vi "Write fsync.vi"(8 "error in (no error)":errorcluster, 10 "enable fsync":bool, 11 "session in":refnum<class "Session.lvclass">) -> (0 "error out":errorcluster, 3 "session out":refnum<class "Session.lvclass">)   [LabVIEW 2020, in "NI_SFTP.lvlib" / "Session.lvclass"]
doc: "Sets whether file data is flushed to disk after successful download or upload."
uses:
  <vilib>/net/SFTP/Session/Session.lvclass
  <vilib>/net/SFTP/Session/Session.lvclass/Session.ctl
  <vilib>/net/SFTP/Session/Is Connected.vi
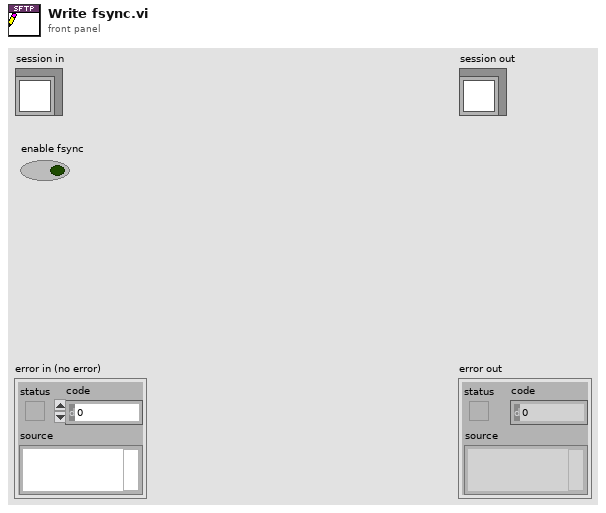
[diagram p1: front panel]
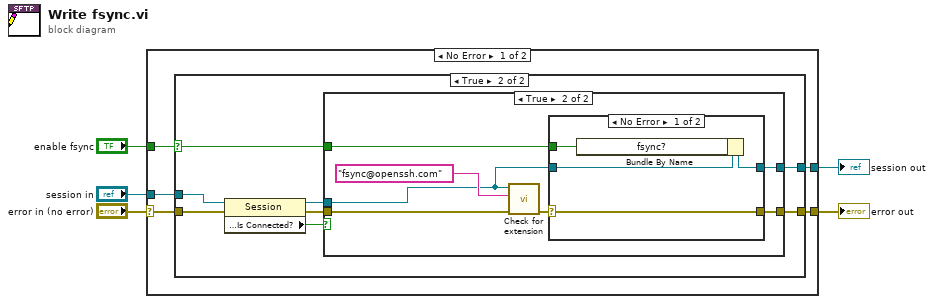
[diagram p0: block diagram]
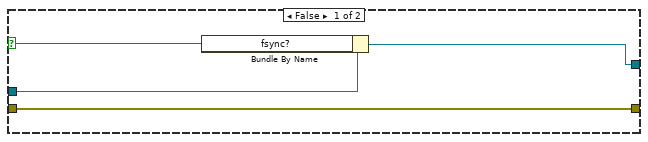
[diagram p2: hidden frame]
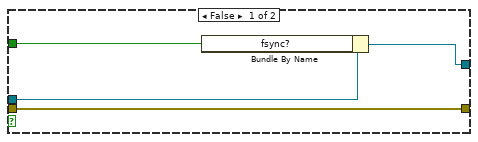
[diagram p3: hidden frame]
diagram:
  n1 = case shown="No Error" "error in (no error)" {
    selector: "error in (no error)" -> [w8 w40]
    tunnel: [w6 w40] -> w4
    tunnel: [w10 w41] -> w2
    tunnel: "session in" -> [w9 w41]
    tunnel: "enable fsync" -> [w7 _]
    frame No Error {
      n2 = case shown="True" w7 {
        selector: w7 -> [w12 w16]
        tunnel: [w13 w22] -> w10
        tunnel: w9 -> [w14 w21]
        tunnel: w8 -> [w11 w20]
        tunnel: [w11 w15] -> w6
        frame False {
          n3 = Bundle By Name(cluster=w14, "fsync?"=w12) -> (w13:refnum<class "Session.lvclass">)
        }
        frame True {
          n4 = property class="Session"(reference=w21, error in=w20) -> (reference out=w17:refnum<class "Session.lvclass">, error out=w18:errorcluster, "Properties:Is Connected?"=w19:bool)
          n5 = case shown="True" w19 {
            tunnel: [w25 w33] -> w22
            tunnel: w18 -> [w24 w32]
            tunnel: w17 -> [w23 w27]
            tunnel: w16 -> [w26 w29]
            tunnel: [w24 w28] -> w15
            frame False {
              n6 = Bundle By Name(cluster=w23, "fsync?"=w26) -> (w25:refnum<class "Session.lvclass">)
            }
            frame True {
              n7 = call <vilib>:"Check for extension.vi"("error in (no error)"=w32, "extension name"="fsync@openssh.com" ("name"), "session in"=w27) -> ("error out"=w30:errorcluster)  [unwired: 8 in]
              n8 = case shown="No Error" w30 {
                selector: w30 -> [w34 w39]
                tunnel: [w37 w38] -> w33
                tunnel: w27 -> [w36 w38]
                tunnel: w29 -> [w35 _]
                tunnel: [w34 w39] -> w28
                frame No Error {
                  n9 = Bundle By Name(cluster=w36, "fsync?"=w35) -> (w37:refnum<class "Session.lvclass">)
                }
                frame Error {
                }
              }
            }
          }
        }
      }
    }
    frame Error {
    }
  }
  "error out" <- w4
  "session out" <- w2
